vi "Network trigger Receiver.vi"() -> ()   [LabVIEW 2020]
uses:
  shared/stop FGV control.ctl
  <vilib>/Utility/tcp.llb/UDP Multicast Read-Only Open.vi
panel:
  out "error out":errorcluster
  out "remote IP":string
  out "IP matching DB subnet":string
  in  "address":string="239.192.5.35"
  in  "receiver port":u16=61000
  in  "stop":bool
  in  "error in (no error)":errorcluster
  out "connection ID":refnum<k16>
  out "No error":errorcluster
  out "2nd udp error":errorcluster
  out "wait time":u32
  out "current time":timestamp
  out "NetTrigger Time Stamp":timestamp
  out "data out 2":string
  out "x-y":dbl
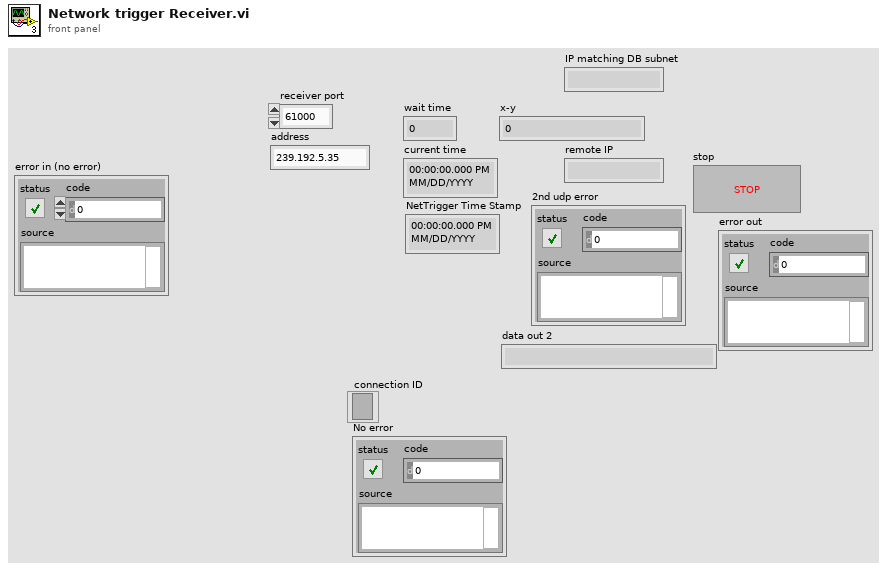
[diagram p1: front panel]
types:
  T1 = enum32{"Invalid", "Standard", "Closed", "Hidden", "Minimized", "Maximized"}
  T2 = typedef "stop FGV control.ctl" = enum16{"Clear", "Write", "Read"}
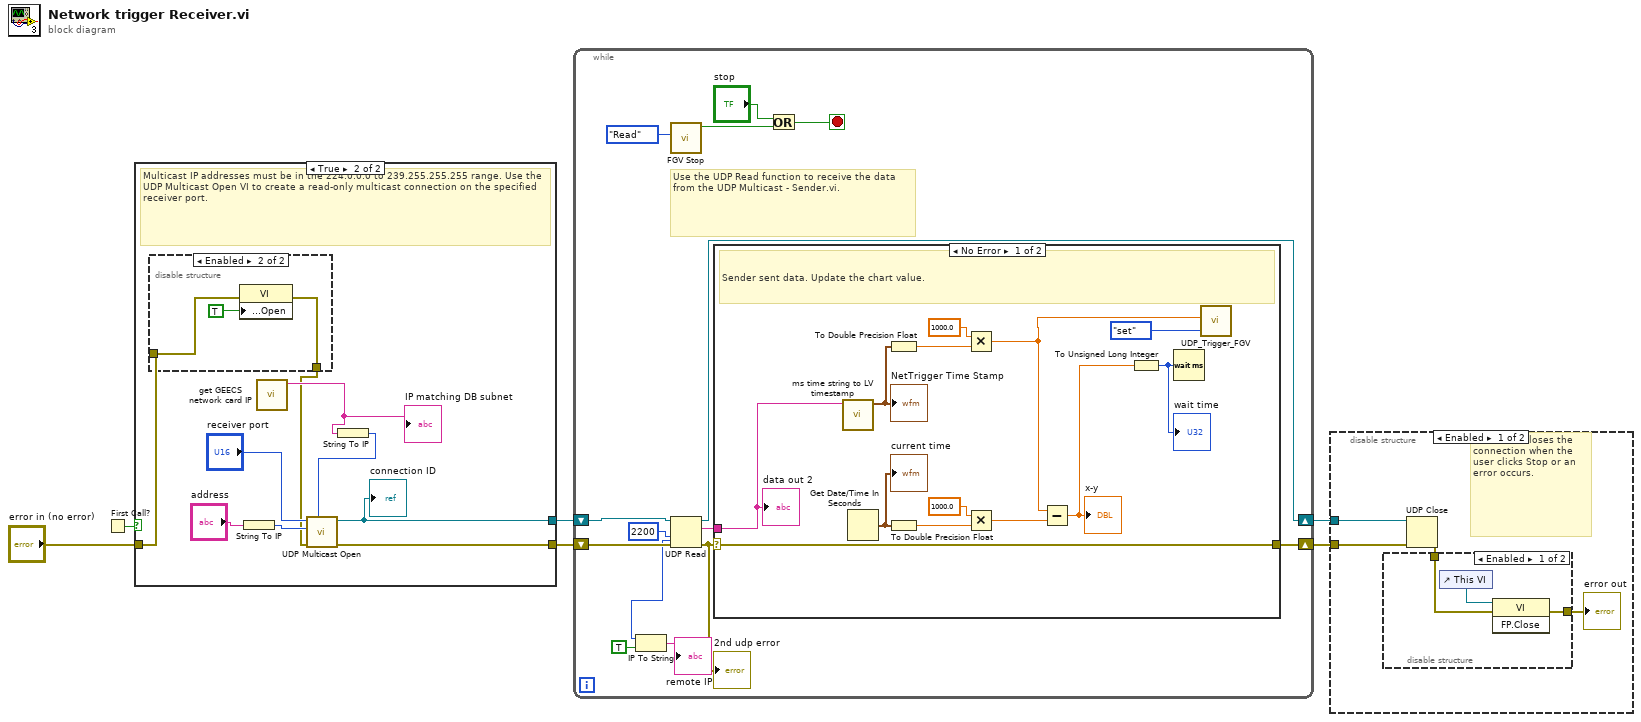
[diagram p0: block diagram]
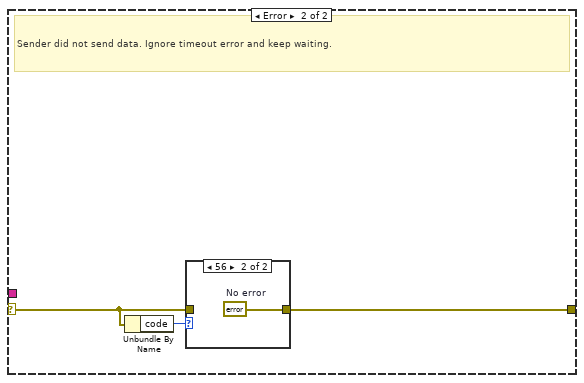
[diagram p2: hidden frame]
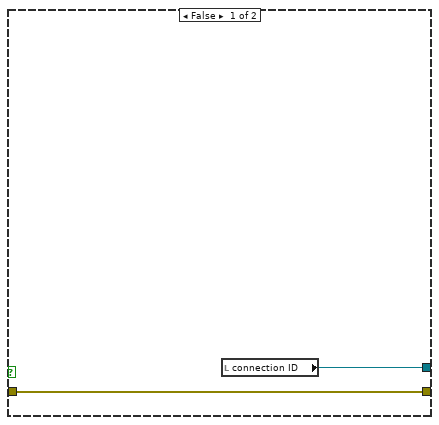
[diagram p4: hidden frame]
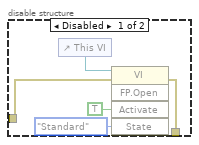
[diagram p5: hidden frame]
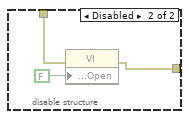
[diagram p6: hidden frame]
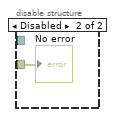
[diagram p7: hidden frame]
diagram:
  n1 = First Call?() -> (First Call?: T/F=w6:bool)
  n2 = case shown="True" w6 {
    tunnel: [w8 w16] -> w3
    tunnel: [w7 w13] -> w2
    tunnel: "error in (no error)" -> [w8 w10]
    frame False {
      n3 = local read "connection ID"() -> (w7:refnum<k16>)
    }
    frame True {
      # "Multicast IP addresses must be in the 224.0.0.0 to 239.255.255.255 range. Use the UDP Multicast Open VI to create a read-only multicast connection on the specified receiver port."
      n4 = disable-structure shown="Enabled" {
        disable-tunnel: w10 -> [w20 w24]
        disable-tunnel: [w19 w23] -> w9
        frame Disabled {
          n5 = control-ref of="This VI"() -> (w22:refnum<vi>)
          n6 = invoke class="VI" method="FP.Open"(reference=w22, error in=w20, "Activate"=TRUE ("Activate?"), "State"=T1."Standard") -> (error out=w19:errorcluster)  [unwired: 1 in, 4 out]
        }
        frame Enabled {
          n7 = property class="VI"(error in=w24, "Front Panel Window:Open"=TRUE) -> (error out=w23:errorcluster)  [unwired: 1 in, 1 out]
        }
      }
      n8 = String To IP(1:"address") -> (0:w14:u32)
      n9 = call "get GEECS network card IP.vi"() -> ("GEECS computer IP"=w11:string)  [unwired: 11 in]
      "IP matching DB subnet" <- w11
      n10 = String To IP(1:w11) -> (0:w12:u32)
      n11 = call-poly <vilib>:"UDP Multicast Open.vi"("net address"=w12, "error in (no error)"=w9, "multicast addr"=w14, "port"="receiver port") -> ("error out"=w16:errorcluster, "connection ID"=w13:refnum<k16>)  [unwired: 5 in, 1 out]
      "connection ID" <- w13
    }
  }
  n12 = while {
    shift-right: [w37] -> w5
    shift-left: w3 -> [w35]
    shift-right: [w36] -> w4
    shift-left: w2 -> [w34]
    stop <- w29 stop-if-true
    # "Use the UDP Read function to receive the data from the UDP Multicast - Sender.vi."
    n13 = call "FGV Stop.vi"("Function"=stop_FGV_control."Read") -> ("stop out"=w30:bool)  [unwired: 9 in, 1 out]
    n14 = UDP Read(connection ID=w34, timeout ms (25000)=2200, 8:w35) -> (data out=w39:string, error out=w33:errorcluster, 3:w36:refnum<k16>, 6:w28:u32)  [unwired: 2 out]
    "2nd udp error" <- w33
    n15 = IP To String(1:TRUE ("dot notation? (F)"), 2:w28) -> (0:→"remote IP":string)
    n16 = case shown="No Error" w33 {
      selector: w33 -> [w52 w53]
      tunnel: w39 -> [w51 _]
      tunnel: [w52 w54] -> w37
      frame No Error {
        # "Sender sent data. Update the chart value."
        n17 = call "ms time string to LV timestamp.vi"("String"=w51) -> ("Time Stamp"=w45:timestamp)  [unwired: 10 in]
        "NetTrigger Time Stamp" <- w45
        n18 = Get Date/Time In Seconds() -> (seconds since 1Jan1904=w50:timestamp)
        "current time" <- w50
        n19 = To Double Precision Float(number=w45) -> (double precision float=w47:dbl)
        n20 = To Double Precision Float(number=w50) -> (double precision float=w48:dbl)
        n21 = Multiply(x=1000.0 ("y"), y=w47) -> (x*y=w40:dbl)
        n22 = Multiply(x=1000.0 ("y"), y=w48) -> (x*y=w44:dbl)
        n23 = Subtract(x=w40, y=w44) -> (x-y=w43:dbl)
        "x-y" <- w43
        n24 = To Unsigned Long Integer(number=w43) -> (unsigned 32bit integer=w42:u32)
        "wait time" <- w42
        n25 = Wait (ms)(milliseconds to wait=w42) -> ()  [unwired: 1 out]
        n26 = call "UDP_Trigger_FGV.vi"("ms timestamp network trigger in"=w40, "command"=enum16{"set", "get", "reset"}."set") -> ()  [unwired: 9 in, 1 out]
        "data out 2" <- w51
      }
      frame Error {
        # "Sender did not send data. Ignore timeout error and keep waiting."
        n27 = Unbundle By Name(w53) -> ("code"=w55:i32)
        n28 = case shown="56" w55 {
          tunnel: w53 -> [w56 _]
          tunnel: [w56 w57] -> w54
          frame Default {
          }
          frame 56 {
            w57 = errorcluster {"status"=FALSE, "code"=0, "source"=""}  # No error
          }
        }
      }
    }
    n29 = Or(x="stop", y=w30) -> (x .or. y?=w29:bool)
  }
  n30 = disable-structure shown="Enabled" {
    disable-tunnel: w4 -> [w61 _]
    disable-tunnel: w5 -> [w60 w68]
    frame Enabled {
      # "UDP Close closes the connection when the user clicks Stop or an error occurs."
      n31 = UDP Close(connection ID=w61, 8:w60) -> (error out=w59:errorcluster)  [unwired: 1 out]
      n32 = disable-structure shown="Enabled" {
        disable-tunnel: w59 -> [w63 w67]
        disable-tunnel: [w62 w65] -> w58
        frame Enabled {
          n33 = control-ref of="This VI"() -> (w64:refnum<vi>)
          n34 = invoke class="VI" method="FP.Close"(reference=w64, error in=w63) -> (error out=w62:errorcluster)  [unwired: 1 in, 2 out]
        }
        frame Disabled {
          n35 = property class="VI"(error in=w67, "Front Panel Window:Open"=FALSE) -> (error out=w65:errorcluster)  [unwired: 1 in, 1 out]
        }
      }
      "error out" <- w58
    }
    frame Disabled {
      "No error" <- w68
    }
  }
